vi "DownsampleStage2.vi"(8 "valid in":bool, 9 "reset":bool, 11 "Element":fxp<+/-,20,16>[](array[numeric])=[0.0, 0.0, 0.0, 0.0]) -> (0 "valid out":bool, 3 "Element":u64, 5 "dout":fxp<+/-,25,19>, 7 "cic valid out":bool)   [LabVIEW 2013]
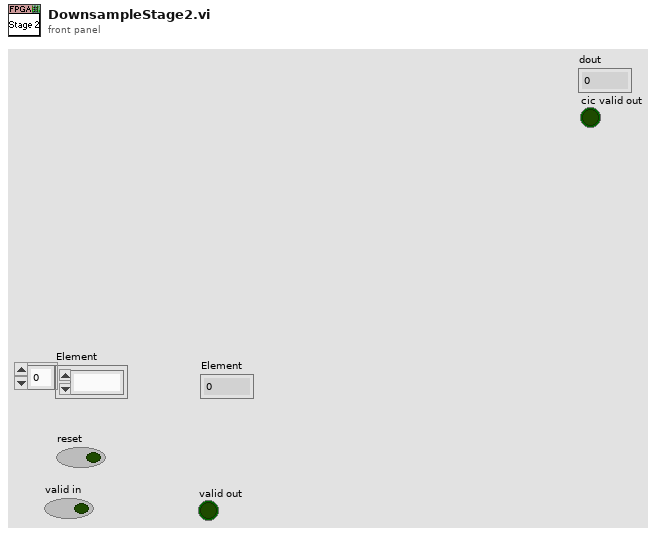
[diagram p1: front panel]
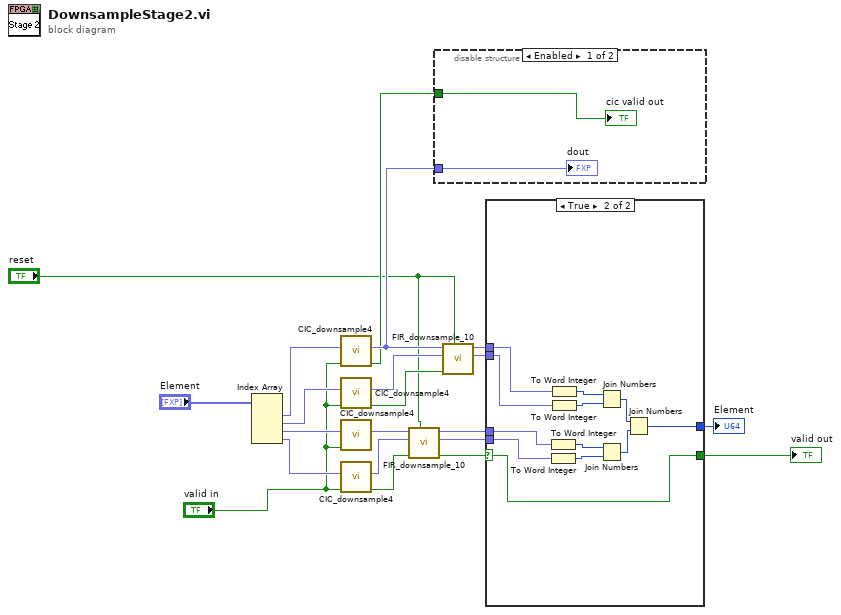
[diagram p0: block diagram]
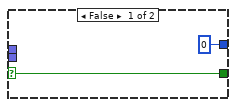
[diagram p3: hidden frame]
diagram:
  n1 = Index Array(array="Element") -> (element #1=w17:fxp<+/-,20,16>, element #2=w18:fxp<+/-,20,16>, element #3=w19:fxp<+/-,20,16>, element #4=w20:fxp<+/-,20,16>)  [unwired: 4 in]
  n2 = call "CIC_downsample4.vi"("valid in"="valid in", "din"=w17) -> ("valid out"=w2:bool, "dout"=w15:fxp<+/-,25,19>)  [unwired: 7 in, 1 out]
  n3 = call "CIC_downsample4.vi"("valid in"="valid in", "din"=w18) -> ("valid out"=w4:bool, "dout"=w16:fxp<+/-,25,19>)  [unwired: 7 in, 1 out]
  n4 = call "CIC_downsample4.vi"("valid in"="valid in", "din"=w19) -> ("dout"=w14:fxp<+/-,25,19>)  [unwired: 7 in, 2 out]
  n5 = call "CIC_downsample4.vi"("valid in"="valid in", "din"=w20) -> ("valid out"=w12:bool, "dout"=w13:fxp<+/-,25,19>)  [unwired: 7 in, 1 out]
  n6 = call "FIR_downsample_10.vi"("reset"="reset", "valid in"=w12, "Q in"=w13, "I in"=w14) -> ("valid out"=w11:bool, "Q out"=w7:fxp<+/-,16,16>, "I out"=w8:fxp<+/-,16,16>)  [unwired: 4 in, 1 out]
  n7 = disable-structure shown="Enabled" {
    disable-tunnel: w15 -> [w23 _]
    disable-tunnel: w2 -> [w22 _]
    frame Enabled {
      "dout" <- w23
      "cic valid out" <- w22
    }
    frame Disabled {
    }
  }
  n8 = call "FIR_downsample_10.vi"("reset"="reset", "valid in"=w4, "Q in"=w16, "I in"=w15) -> ("Q out"=w9:fxp<+/-,16,16>, "I out"=w10:fxp<+/-,16,16>)  [unwired: 4 in, 2 out]
  n9 = case shown="True" w11 {
    selector: w11 -> [w24 w26]
    tunnel: w10 -> [_ w31]
    tunnel: w9 -> [_ w30]
    tunnel: w8 -> [_ w29]
    tunnel: w7 -> [_ w28]
    tunnel: [u64 0 w27] -> w6
    tunnel: [w24 w26] -> w5
    frame False {
    }
    frame True {
      n10 = To Word Integer(number=w29) -> (16bit integer=w35:i16)
      n11 = To Word Integer(number=w28) -> (16bit integer=w34:i16)
      n12 = To Word Integer(number=w31) -> (16bit integer=w36:i16)
      n13 = To Word Integer(number=w30) -> (16bit integer=w37:i16)
      n14 = Join Numbers(hi=w36, lo=w37) -> ((hi.lo)=w33:u32)
      n15 = Join Numbers(hi=w35, lo=w34) -> ((hi.lo)=w32:u32)
      n16 = Join Numbers(hi=w33, lo=w32) -> ((hi.lo)=w27:u64)
    }
  }
  "Element" <- w6
  "valid out" <- w5
